vi "Save Data.vi"(4 "error in (no error)":errorcluster, 6 "My Name":T1, 7 "History Data":dbl[](array[numeric])) -> (0 "error out":errorcluster)   [LabVIEW 2015, in "Startup Processes.lvlib"]
uses:
  Startup Processes.lvlib
  _typedefs/Subpanel Names.ctl
  <vilib>/Utility/sysdir.llb/System Directory Type.ctl
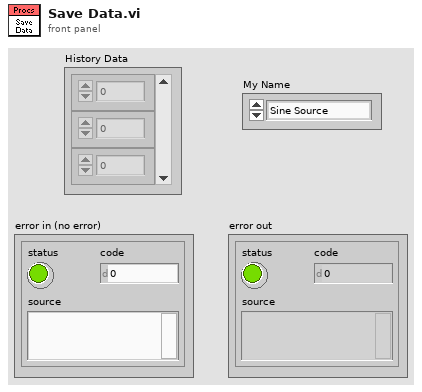
[diagram p1: front panel]
types:
  T1 = typedef "Startup Processes.lvlib/Subpanel Names.ctl" = enum16{"Sine Source", "Ramp Source", "Hen House TC", "Dog House TC", "Out House TC"}
  T2 = typedef "System Directory Type.ctl" = i32
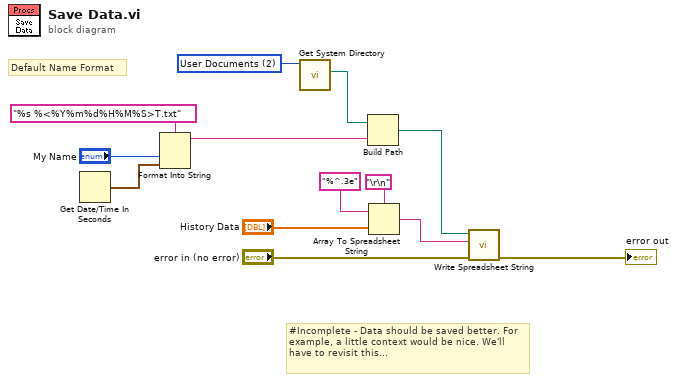
[diagram p0: block diagram]
diagram:
  w2 = T2 2 items=["User Home"=0, "User Desktop"=1, "User Documents"=2, "User Application Data"=3, "User Preferences"=4, "User Temporary"=5, "Public Documents"=6, "Public Application Data"=7, "Public Preferences"=8, "Public Cache"=13, "System Core Libraries"=9, "System Installed Libraries"=10, "Application Files"=11, "Boot Volume Root"=12] ("system directory type")
  # "Default Name Format"
  # "#Incomplete - Data should be saved better. For example, a little context would be nice. We'll have to revisit this..."
  n1 = Get Date/Time In Seconds() -> (seconds since 1Jan1904=w9:timestamp)
  n2 = Format Into String(format string="%s %<%Y%m%d%H%M%S>T.txt", "My Name", w9) -> (resulting string=w5:string)  [unwired: 2 in, 1 out]
  n3 = call <vilib>:"Get System Directory.vi"("system directory type"=w2) -> ("system directory"=w3:path)  [unwired: 10 in]
  n4 = Build Path(base path=w3, name or relative path=w5) -> (appended path=w4:path)
  n5 = Array To Spreadsheet String(delimiter (Tab)="\r\n", array="History Data", 3:"%^.3e" ("format (%.3f)")) -> (spreadsheet string=w6:string)
  n6 = call <vilib>:"Write Spreadsheet String.vi"("error in"="error in (no error)", "spreadsheet string"=w6, "file path (dialog if empty)"=w4) -> ("error out"=→"error out":errorcluster)  [unwired: 7 in, 1 out]
